vi "not_even_an_event_structure.vi"() -> ()   [LabVIEW 2023]
panel:
  in  "Check":bool
  out "Liczba iteracji":i32
  out "Array":bool[](array[boolean])
  in  "Boolean 8":bool=TRUE
  in  "stop":bool
  in  "Enum":enum16{"XOR", "OR", "AND"}(ring)
  out "Boolean 24":bool
  out "Boolean 23":bool
  out "Boolean 22":bool
  out "Boolean 21":bool
  out "Boolean 20":bool
  out "Boolean 19":bool
  out "Boolean 18":bool
  out "Boolean 17":bool
  in  "Boolean 16":bool
  in  "Boolean 15":bool
  in  "Boolean 14":bool
  in  "Boolean 13":bool
  in  "Boolean 12":bool
  in  "Boolean 11":bool
  in  "Boolean 10":bool
  in  "Boolean 9":bool
  in  "Boolean 7":bool
  in  "Boolean 6":bool
  in  "Boolean 5":bool
  in  "Boolean 4":bool
  in  "Boolean 3":bool
  in  "Boolean 2":bool
  in  "Boolean":bool
  # "Bajt 1"
  # "Bajt 2"
  # "Wynik"
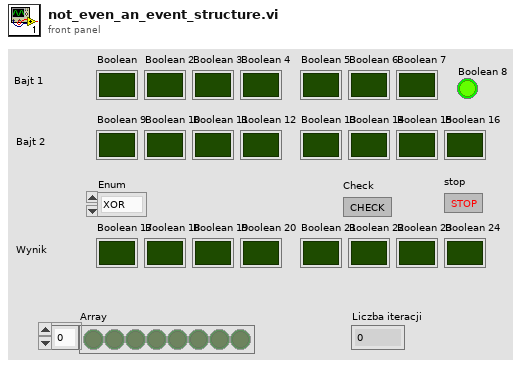
[diagram p1: front panel]
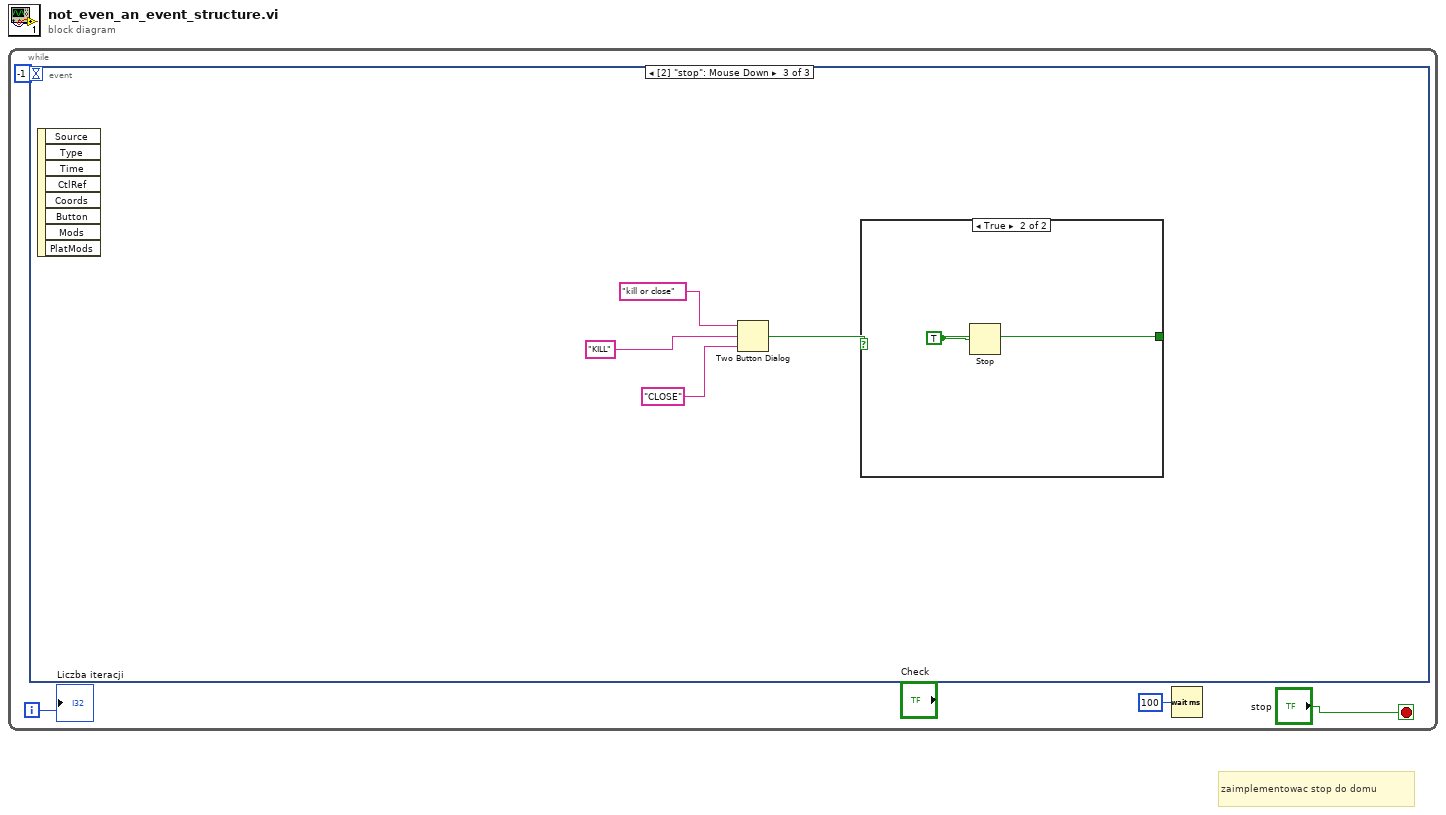
[diagram p0: block diagram]
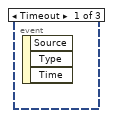
[diagram p2: hidden frame]
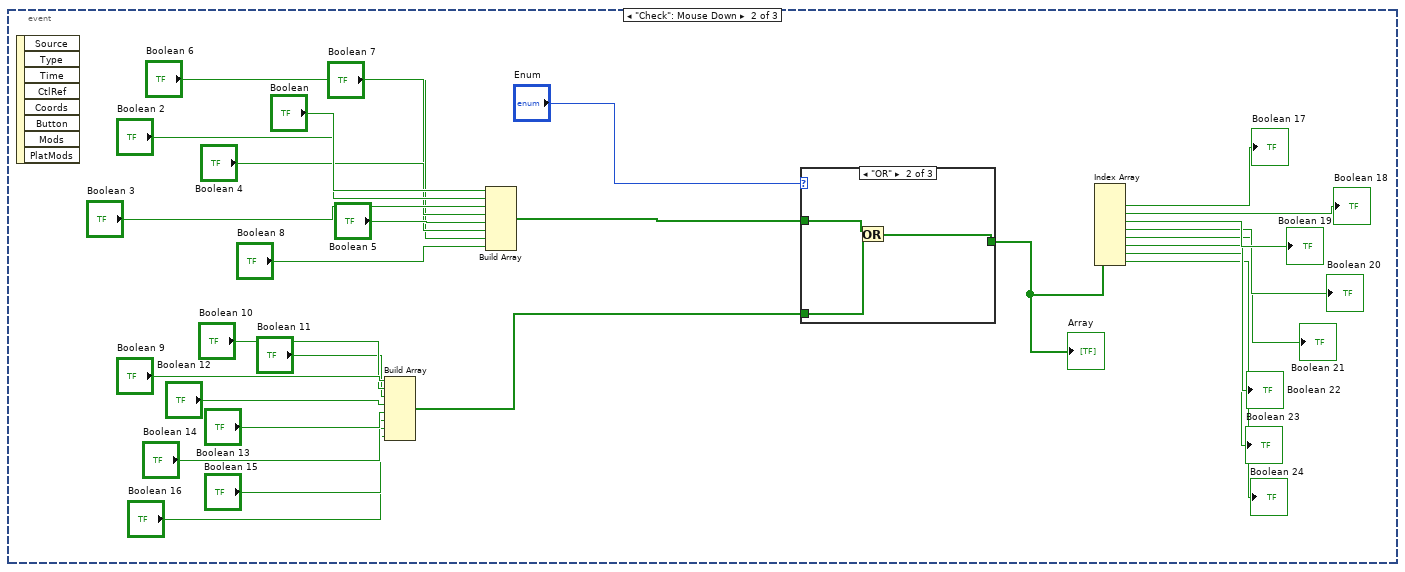
[diagram p3: hidden frame]
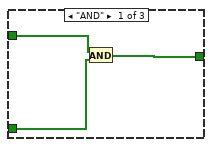
[diagram p4: hidden frame]
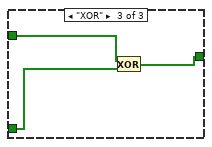
[diagram p5: hidden frame]
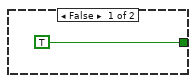
[diagram p6: hidden frame]
diagram:
  # "zaimplementowac stop do domu"
  n1 = while {
    i -> [w4]
    stop <- "stop" stop-if-true
    n2 = event shown="[2] \"stop\": Mouse Down" {
      selector: _ -> [_ _ _]
      dyn-events: _ -> [_ _ _]
      timeout: -1 -> [_ _ _]
      event Timeout {
        n3 = event-data() -> ()  [unwired: 1 in, 3 out]
      }
      event "Check": Mouse Down {
        n4 = event-data() -> ()  [unwired: 1 in, 8 out]
        n5 = Build Array("Boolean 9", "Boolean 10", "Boolean 11", "Boolean 12", "Boolean 13", "Boolean 14", "Boolean 15", "Boolean 16") -> (w15:bool[])
        n6 = Build Array("Boolean", "Boolean 2", "Boolean 3", "Boolean 4", "Boolean 5", "Boolean 6", "Boolean 7", "Boolean 8") -> (w14:bool[])
        n7 = case shown="\"OR\"" "Enum" {
          tunnel: w15 -> [w34 w37 w40]
          tunnel: w14 -> [w35 w38 w41]
          tunnel: [w33 w36 w39] -> w13
          frame "AND" {
            n8 = And(x=w35, y=w34) -> (x .and. y?=w33:bool[])
          }
          frame "OR" {
            n9 = Or(x=w38, y=w37) -> (x .or. y?=w36:bool[])
          }
          frame "XOR" {
            n10 = Exclusive Or(1:w40, 2:w41) -> (0:w39:bool[])
          }
        }
        "Array" <- w13
        n11 = Index Array(array=w13) -> (element #1=→"Boolean 17":bool, element #2=→"Boolean 18":bool, element #3=→"Boolean 19":bool, element #4=→"Boolean 20":bool, element #5=→"Boolean 21":bool, element #6=→"Boolean 22":bool, element #7=→"Boolean 23":bool, element #8=→"Boolean 24":bool)  [unwired: 8 in]
      }
      event "stop": Mouse Down {
        n12 = event-data() -> ()  [unwired: 1 in, 8 out]
        n13 = Two Button Dialog(message="kill or close", 1:"CLOSE" ("F button name (\"Cancel\")"), 2:"KILL" ("T button name (\"OK\")")) -> (T button?=w45:bool)
        n14 = case shown="True" w45 {
          tunnel: [TRUE w47] -> _
          frame False {
          }
          frame True {
            w47 = TRUE
            n15 = Stop(stop? (T)=w47) -> ()
          }
        }
      }
    }
    n16 = Wait (ms)(milliseconds to wait=u32 100) -> ()  [unwired: 1 out]
    "Liczba iteracji" <- w4
  }
